vi "Template Encode Decode File.vi"(8 "String to decode":string, 11 "String to encode":string) -> (0 "decoded String":string, 3 "encoded String":string)   [LabVIEW 2011]
panel:
  out "unsigned byte array":u8[](array[numeric])
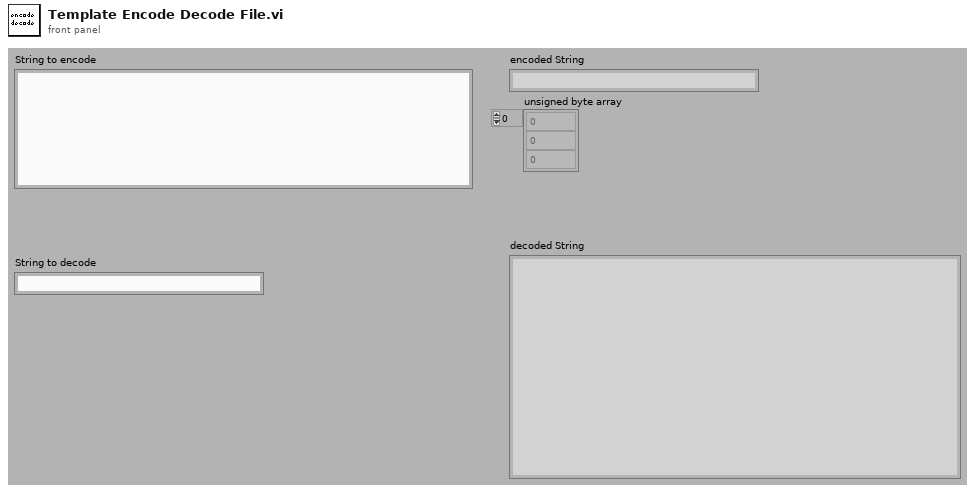
[diagram p1: front panel]
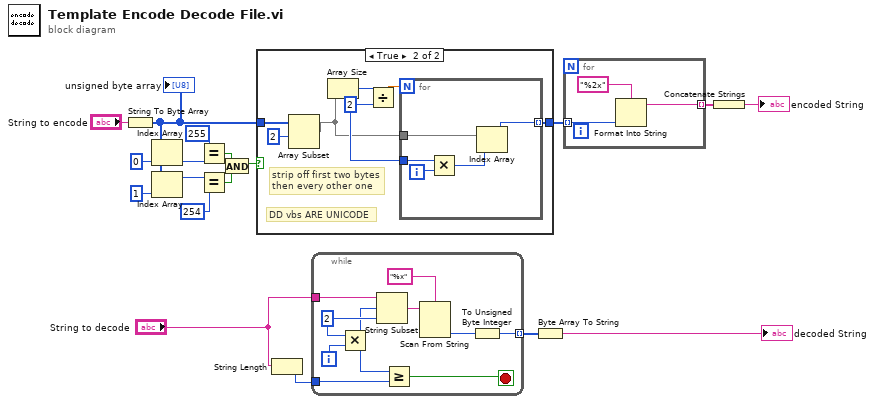
[diagram p0: block diagram]
diagram:
  n1 = String To Byte Array(string="String to encode") -> (unsigned byte array=w10:u8[])
  "unsigned byte array" <- w10
  n2 = Index Array(array=w10, index=0) -> (element=w4:u8)
  n3 = Index Array(array=w10, index=1) -> (element=w3:u8)
  n4 = Equal?(x=u8 255 ("index"), y=w4) -> (x = y?=w7:bool)
  n5 = Equal?(x=w3, y=u8 254 ("index")) -> (x = y?=w5:bool)
  n6 = And(x=w7, y=w5) -> (x .and. y?=w6:bool)
  n7 = case shown="True" w6 {
    tunnel: w10 -> [w19 w22]
    tunnel: [w19 w24] -> w11
    frame False {
    }
    frame True {
      w23 = 2 ("y")
      # "DD vbs ARE UNICODE"
      # "strip off first two bytes\nthen every other one"
      n8 = Array Subset(array=w22, index=2) -> (w20:u8[])  [unwired: 1 in]
      n9 = Array Size(array=w20) -> (size(s)=w26:i32)
      n10 = Divide(x=w26, y=w23) -> (x/y=w25:dbl)
      n11 = for {
        N: w25 -> [_]
        tunnel: w20 -> [w31]
        tunnel: [w30] -> w24 mode=indexing
        tunnel: w23 -> [w28]
        i -> [w29]
        n12 = Multiply(x=w28, y=w29) -> (x*y=w27:i32)
        n13 = Index Array(array=w31, index=w27) -> (element=w30:u8)
      }
    }
  }
  n14 = String Length(string="String to decode") -> (length=w14:i32)
  n15 = while {
    tunnel: "String to decode" -> [w41]
    tunnel: [w35] -> w16 mode=indexing
    tunnel: w14 -> [w34]
    i -> [w40]
    stop <- w33 stop-if-true
    w39 = 2 ("length (rest)")
    n16 = Multiply(x=w39, y=w40) -> (x*y=w32:i32)
    n17 = String Subset(string=w41, offset (0)=w32, length (rest)=w39) -> (substring=w38:string)
    n18 = Greater Or Equal?(x=w32, y=w34) -> (x >= y?=w33:bool)
    n19 = Scan From String(format string="%x", input string=w38) -> (output 1=w36:i32)  [unwired: 2 in, 4 out]
    n20 = To Unsigned Byte Integer(number=w36) -> (unsigned 8bit integer=w35:u8)
  }
  n21 = Byte Array To String(unsigned byte array=w16) -> (string=→"decoded String":string)
  n22 = for {
    tunnel: w11 -> [w44] mode=indexing
    tunnel: [w42] -> w17 mode=indexing
    n23 = Format Into String(format string="%2x", w44) -> (resulting string=w42:string)  [unwired: 2 in, 1 out]
  }
  n24 = Concatenate Strings(w17) -> (→"encoded String":string)
